vi "SaveWaveformsASCII.vi"(4 "Transpose":bool=TRUE, 5 "Format":string="%.6g", 6 "Deafault channel name prefix":string="CH", 7 "Channel name attribute":string="NI_ChannelName", 8 "Error In":errorcluster, 9 "Save column names":bool=TRUE, 10 "Waveforms":waveform(dbl)[](array[waveform]), 11 "File":path) -> (0 "Error Out":errorcluster, 3 "File out":path)   [LabVIEW 2015]
uses:
  <vilib>/Utility/file.llb/Write Delimited Spreadsheet (DBL).vi
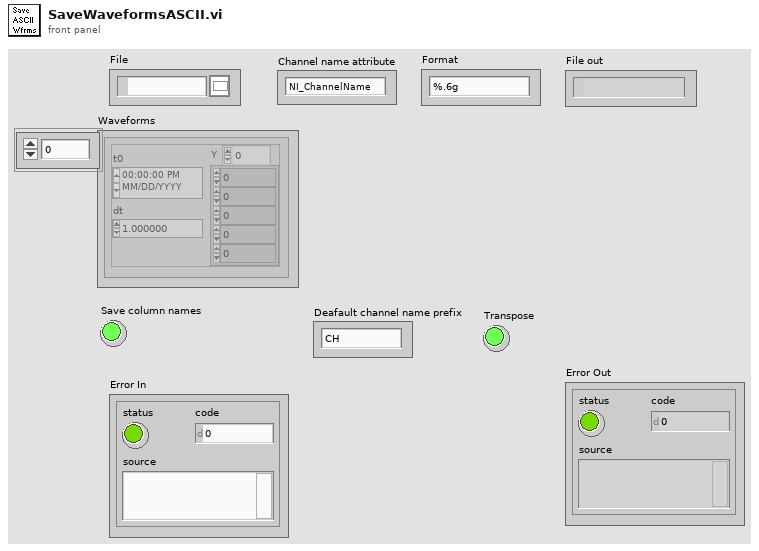
[diagram p1: front panel]
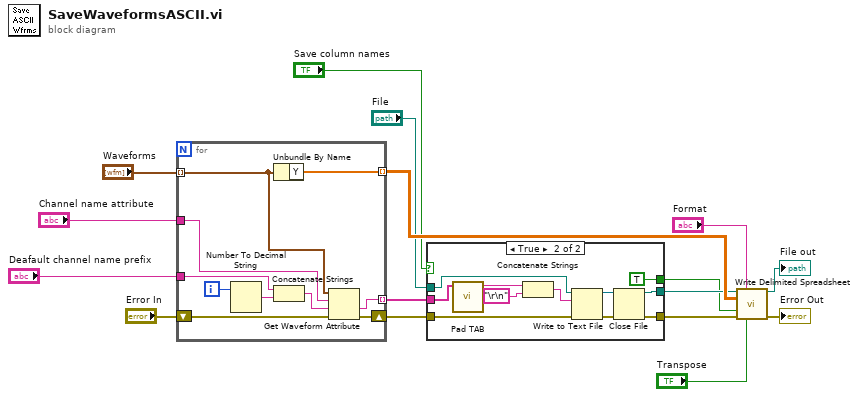
[diagram p0: block diagram]
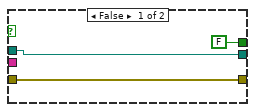
[diagram p2: hidden frame]
diagram:
  n1 = for {
    tunnel: "Waveforms" -> [w25] mode=indexing
    tunnel: [w26] -> w11 mode=indexing
    tunnel: "Channel name attribute" -> [w24]
    tunnel: "Deafault channel name prefix" -> [w23]
    shift-right: [w21] -> w13
    shift-left: "Error In" -> [w22]
    tunnel: [w17] -> w14 mode=indexing
    i -> [w19]
    n2 = Number To Decimal String(number=w19) -> (decimal integer string=w18:string)  [unwired: 1 out]
    n3 = Unbundle By Name(w25) -> ("Y"=w26:dbl[])
    n4 = Concatenate Strings(w23, w18) -> (w20:string)
    n5 = Get Waveform Attribute(4:w22, 5:w20, 6:w24, 7:w25) -> (0:w21:errorcluster, 1:w17:string)  [unwired: 2 out]
  }
  n6 = case shown="True" "Save column names" {
    tunnel: [FALSE ("append to file? (new file:F)") TRUE] -> w4
    tunnel: [w27 w34] -> w12
    tunnel: w14 -> [_ w38]
    tunnel: [w28 w32] -> w10
    tunnel: w13 -> [w27 w31]
    tunnel: "File" -> [w28 w30]
    frame False {
    }
    frame True {
      n7 = call "Pad TAB.vi"("Input String Array"=w38) -> ("Output String"=w39:string)  [unwired: 1 in, 9 out]
      n8 = Concatenate Strings(w39, "\r\n") -> (w37:string)
      n9 = Write to Text File(file (use dialog)=w30, text=w37, error in=w31) -> (refnum out=w33:refnum<file>, error out=w35:errorcluster)  [unwired: 2 out]
      n10 = Close File(refnum=w33, error in=w35) -> (path=w32:path, error out=w34:errorcluster)
    }
  }
  n11 = call-poly <vilib>:"Write Delimited Spreadsheet.vi"("file path (dialog if empty)"=w10, "format (%.3f)"="Format", "2D data"=w11, "append to file? (F)"=w4, "error in (no error)"=w12, "transpose? (F)"="Transpose") -> ("new file path (Not A Path if cancelled)"=→"File out":path, "error out"=→"Error Out":errorcluster)  [unwired: 8 in]
